vi "dfd_Validate WordLen.vi"(8 "error in (no error)":errorcluster, 10 "wl":i16) -> (0 "error out":errorcluster, 2 "dup wl":i16)   [LabVIEW 2017, in "NI_DigFilter_FXP.lvlib"]
uses:
  <vilib>/addons/Digital Filter Design/NI_DigFilter_FXP.lvlib
  <vilib>/addons/Digital Filter Design/_Misc.llb/dfd_Error Handlers (Single).vi
  <vilib>/addons/Digital Filter Design/NI_DigFilterLicensed.lvlib
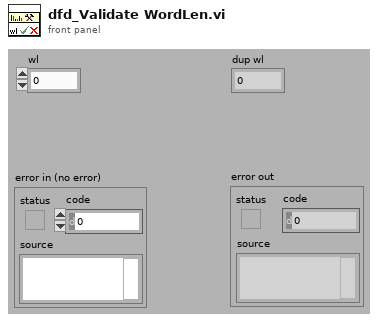
[diagram p1: front panel]
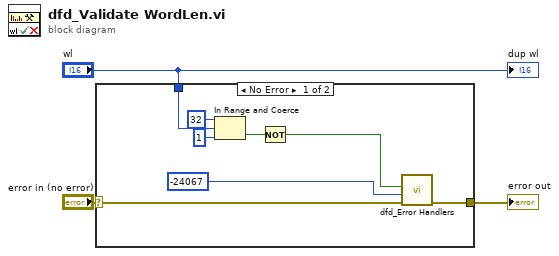
[diagram p0: block diagram]
diagram:
  n1 = case shown="No Error" "error in (no error)" {
    selector: "error in (no error)" -> [w5 w12]
    tunnel: [w4 w12] -> w2
    tunnel: "wl" -> [w11 _]
    frame No Error {
      n2 = In Range and Coerce(upper limit=i16 32, x=w11, lower limit=i16 1) -> (In Range?=w7:bool)  [unwired: 1 out]
      n3 = Not(x=w7) -> (.not. x?=w6:bool)
      n4 = call-poly <vilib>:"dfd_Error Handlers.vi"("error in (no error)"=w5, "error code"=-24067 ("ERR_MRATE_WL_OUT_OF_RANGE"), "condition failed?"=w6) -> ("error out"=w4:errorcluster)  [unwired: 8 out]
    }
    frame Error {
    }
  }
  "error out" <- w2
  "dup wl" <- "wl"
